vi "Session Client FGV.vi"(8 "error in":errorcluster) -> (0 "error out":errorcluster)   [LabVIEW 2020, in "MeasurementLink Session Management Client Wrapper.lvlib"]
uses:
  MeasurementLink Session Management Client Wrapper.lvlib
  Action.ctl
  <vilib>/gRPC/LabVIEW gRPC Library/Shared/grpcId.ctl
  MeasurementLink Measurement Server/MeasurementLink Measurement Server.lvlib
  MeasurementLink Discovery Client/MeasurementLink Discovery Client.lvlib
  MeasurementLink Session Management Client/MeasurementLink Session Management Client.lvlib
  <vilib>/gRPC/LabVIEW gRPC Library/grpc-lvsupport-release.lvlib
panel:
  in  "action":T1
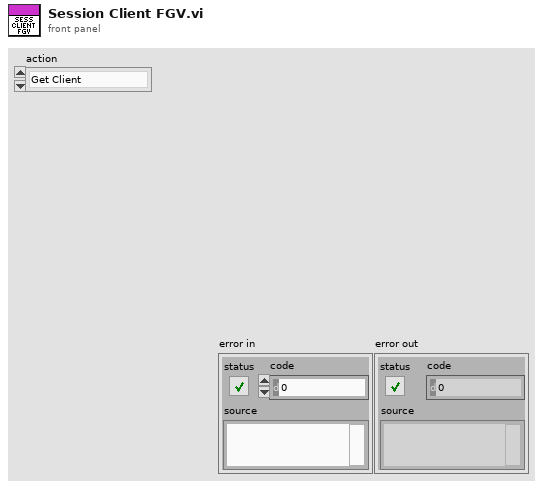
[diagram p1: front panel]
types:
  T1 = typedef "Action.ctl" = enum16{"Get Client", "Destroy Client"}
  T2 = typedef "grpc-lvsupport-release.lvlib/grpcId.ctl" = u64
  T3 = typedef "MeasurementLink Discovery Client.lvlib/ni_measurementlink_discovery_v1_ServiceLocation.ctl" = cluster{"location":string, "insecure_port":string, "ssl_authenticated_port":string}
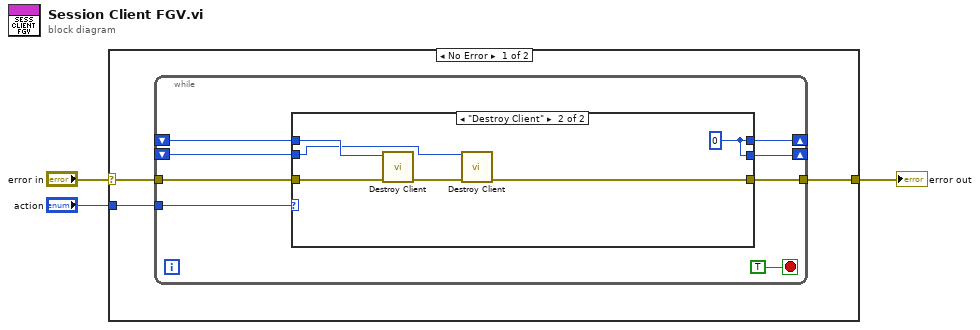
[diagram p0: block diagram]
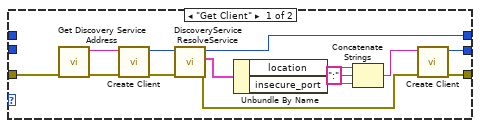
[diagram p2: hidden frame]
diagram:
  n1 = case shown="No Error" "error in" {
    selector: "error in" -> [w5 w35]
    tunnel: [w4 w35] -> w2
    tunnel: "action" -> [w6 _]
    frame No Error {
      n2 = while {
        tunnel: w6 -> [w13]
        tunnel: w5 -> [w12]
        shift-right: [w11] -> _
        shift-left: _ -> [w10]
        tunnel: [w9] -> w4
        shift-right: [w8] -> _
        shift-left: _ -> [w7]
        stop <- TRUE stop-if-true
        n3 = case shown="\"Destroy Client\"" w13 {
          tunnel: w12 -> [w26 w33]
          tunnel: [w20 w29] -> w11
          tunnel: w10 -> [_ w34]
          tunnel: [w16 w30] -> w9
          tunnel: [w15 w29] -> w8
          tunnel: w7 -> [_ w31]
          frame "Get Client" {
            n4 = call "Get Discovery Service Address.vi"("error in"=w26) -> ("error out"=w28:errorcluster, "address"=w27:string)  [unwired: 9 in]
            n5 = call "Create Client.vi"("error in"=w28, "address"=w27) -> ("error out"=w22:errorcluster, "gRPC ID Out"=w21:T2)  [unwired: 8 in]
            n6 = call "DiscoveryService ResolveService.vi"("error in"=w22, "gRPC ID"=w21) -> ("error out"=w17:errorcluster, "Response Data"=w19:T3, "gRPC ID out"=w20:T2)  [unwired: 7 in]
            n7 = Unbundle By Name(w19) -> ("location"=w25:string, "insecure_port"=w24:string)
            n8 = Concatenate Strings(w25, ":" ("string"), w24) -> (w18:string)
            n9 = call "Create Client.vi"("error in"=w17, "address"=w18) -> ("error out"=w16:errorcluster, "gRPC ID Out"=w15:T2)  [unwired: 8 in]
          }
          frame "Destroy Client" {
            w29 = T2 0 ("gRPC ID out")
            n10 = call "Destroy Client.vi"("error in"=w33, "gRPC ID"=w34) -> ("error out"=w32:errorcluster)  [unwired: 9 in]
            n11 = call "Destroy Client.vi"("error in"=w32, "gRPC ID"=w31) -> ("error out"=w30:errorcluster)  [unwired: 9 in]
          }
        }
      }
    }
    frame Error {
    }
  }
  "error out" <- w2
